vi "pp2_cam_writeImage.vi"(10 "File Path":path, 11 "Image":T1) -> ()   [LabVIEW 2013]
uses:
  <vilib>/vision/Image Controls.llb/IMAQ Image.ctl
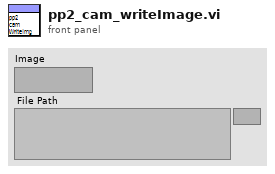
[diagram p1: front panel]
types:
  T1 = typedef "IMAQ Image.ctl" = refnum<image>
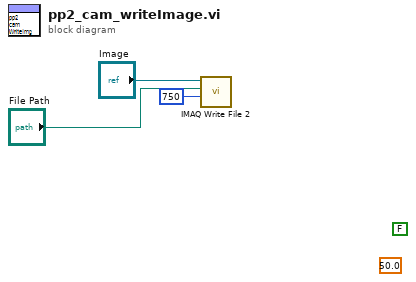
[diagram p0: block diagram]
diagram:
  (unwired) sgl 50.0 ("Compression Ratio")
  (unwired) FALSE ("Lossless? (true)")
  n1 = call-poly "IMAQ Write File 2"("Image Quality"=u32 750, "File Path"="File Path", "Image"="Image") -> ()  [unwired: 7 in, 2 out]
